vi "Get_Each_channel_reference_samplingdata.vi"(0 "SPU":refnum<k24>, 1 "STSProcess.ILSTS":refnum<k24>, 2 "Refdata_struct":refnum<k24>[](array[refnum]), 5 "Ref_monitordata_struct":refnum<k24>[](array[refnum]), 7 "MPM":refnum<k24>[](array[refnum]), 9 "ChannelNumber":i32, 11 "错误输入（无错误）":errorcluster, 12 "TSL":refnum<k24>, 13 "SlotNumber":i32, 14 "MPMNumber":i32) -> (6 "ILSTS out":refnum<k24>, 15 "error out":errorcluster)   [LabVIEW 2017]
doc: "Get logging reference data & add in"
uses:
  D:/test/ILSTS/LV_IL/LV_IL_Sample_x86/DLL/STSProcess.dll
  DLL/STSProcess.dll
  D:/test/ILSTS/LV_IL/LV_IL_Sample_x86/DLL/InstrumentDLL.dll
  DLL/InstrumentDLL.dll
  Share/PowerMonitorType.vi
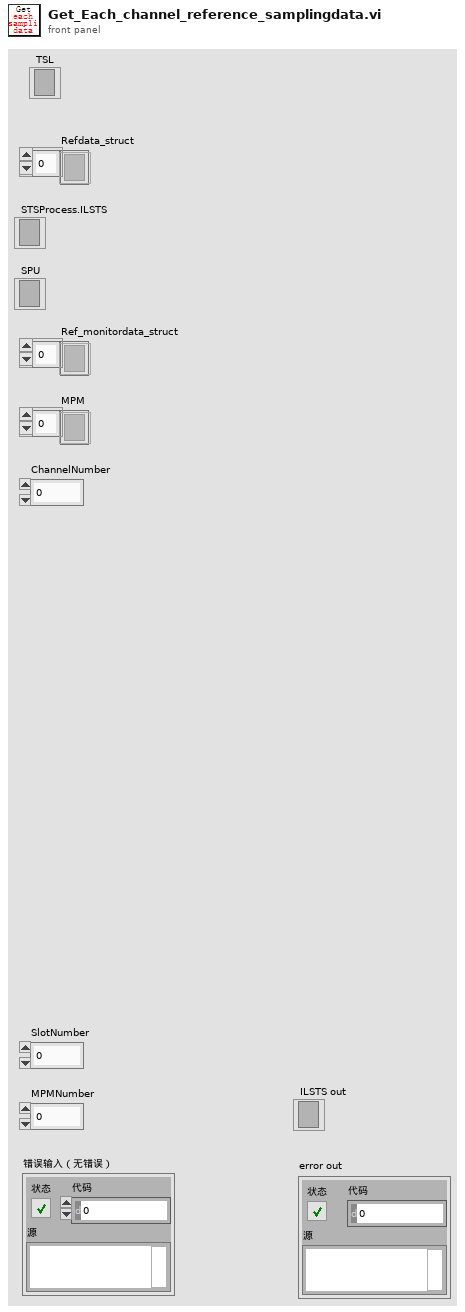
[diagram p1: front panel]
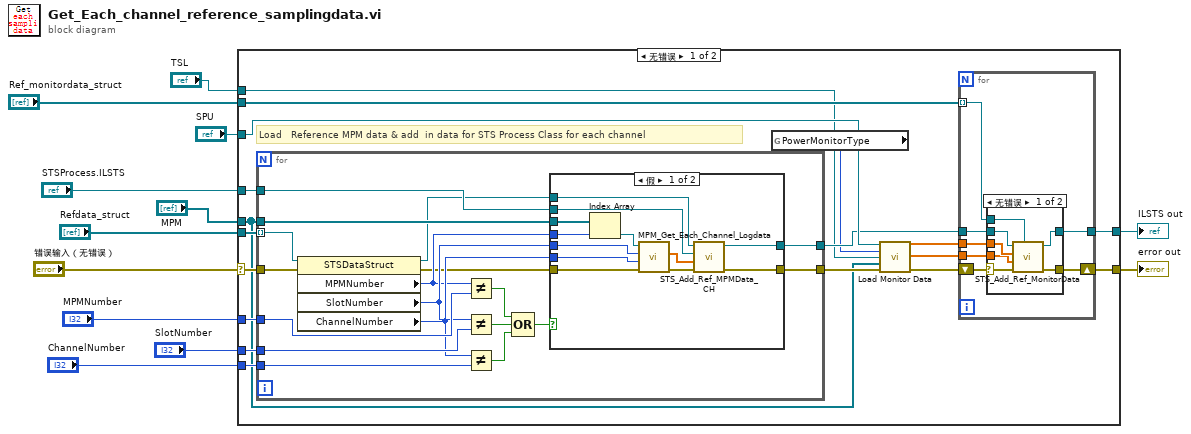
[diagram p0: block diagram]
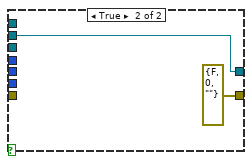
[diagram p3: hidden frame]
diagram:
  n1 = case shown="无错误" "错误输入（无错误）" {
    selector: "错误输入（无错误）" -> [w19 w80]
    tunnel: "STSProcess.ILSTS" -> [w17 w79]
    tunnel: "Ref_monitordata_struct" -> [w27 _]
    tunnel: "SPU" -> [w26 _]
    tunnel: "MPM" -> [w13 _]
    tunnel: "ChannelNumber" -> [w24 _]
    tunnel: "SlotNumber" -> [w23 _]
    tunnel: "MPMNumber" -> [w22 _]
    tunnel: "Refdata_struct" -> [w21 _]
    tunnel: [w20 w80] -> w4
    tunnel: [w18 w79] -> w2
    tunnel: "TSL" -> [w14 _]
    frame No Error {
      # "Load　Reference MPM data & add  in data for STS Process Class for each channel"
      n2 = for {
        tunnel: w21 -> [w52] mode=indexing
        tunnel: w22 -> [w64]
        tunnel: w23 -> [w63]
        tunnel: w24 -> [w62]
        tunnel: w13 -> [w55]
        tunnel: w17 -> [w53]
        tunnel: [w51] -> w25
        tunnel: w19 -> [w49]
        tunnel: [w47] -> w16
        n3 = property on="属性节点" class="STSDataStruct"(reference=w52, error in=w49) -> (reference out=w48:refnum<k24>, error out=w50:errorcluster, "MPMNumber"=w54:i32, "SlotNumber"=w57:i32, "ChannelNumber"=w56:i32)
        n4 = Not Equal?(x=w54, y=w64) -> (x != y?=w61:bool)
        n5 = Not Equal?(x=w57, y=w63) -> (x != y?=w60:bool)
        n6 = Not Equal?(x=w56, y=w62) -> (x != y?=w59:bool)
        n7 = Compound Arithmetic op=OR ("复合运算")(w61, w60, w59) -> (w58:bool)
        n8 = case shown="假" w58 {
          tunnel: w57 -> [w76 _]
          tunnel: w56 -> [w75 _]
          tunnel: w55 -> [w74 _]
          tunnel: w54 -> [w72 _]
          tunnel: w53 -> [w71 w77]
          tunnel: w48 -> [w70 _]
          tunnel: [w67 errorcluster {"status"=FALSE, "code"=0, "source"=""} ("错误输出")] -> w51
          tunnel: w50 -> [w66 _]
          tunnel: [w65 w77] -> w47
          frame False {
            n9 = Index Array(array=w74, index=w72) -> (element=w73:refnum<k24>)
            n10 = call "MPM_Get_Each_Channel_Logdata.vi"("error in (no error)"=w66, "channelNumber"=w75, "moduleNumber"=w76, ".NET Reference in"=w73) -> ("error out"=w68:errorcluster, "data out"=w69:sgl[])  [unwired: 5 in, 1 out]
            n11 = call "STS_Add_Ref_MPMData_CH.vi"("错误输入（无错误）"=w68, "data"=w69, "STSProcess.ILSTS"=w71, "Setting"=w70) -> ("错误输出"=w67:errorcluster, "ILSTS"=w65:refnum<k24>)  [unwired: 6 in]
          }
          frame True {
          }
        }
      }
      n12 = global read "PowerMonitorType.vi" "PowerMonitorType"() -> (w15:enum16{"DAQ", "MPM_220", "TSL_LOGG"})
      n13 = call "Load Monitor Data.vi"("SPU"=w26, "PowerMonitorType"=w15, "TSL"=w14, "MPM"=w13, "error in (no error)"=w25) -> ("trigger"=w29:sgl[], "monitor"=w30:sgl[], "error out"=w28:errorcluster)  [unwired: 8 in]
      n14 = for {
        tunnel: w27 -> [w36] mode=indexing
        tunnel: w16 -> [w37]
        tunnel: w29 -> [w35]
        tunnel: w30 -> [w34]
        shift-right: [w32] -> w20
        shift-left: w28 -> [w33]
        tunnel: [w31] -> w18
        n15 = case shown="无错误" w33 {
          selector: w33 -> [w40 w46]
          tunnel: w37 -> [w44 w45]
          tunnel: w36 -> [w43 _]
          tunnel: w35 -> [w42 _]
          tunnel: w34 -> [w41 _]
          tunnel: [w39 w46] -> w32
          tunnel: [w38 w45] -> w31
          frame No Error {
            n16 = call "STS_Add_Ref_MonitorData.vi"("setting"=w43, "错误输入（无错误）"=w40, "monitorData"=w41, "triggerIndex"=w42, "STSProcess.ILSTS"=w44) -> ("错误输出"=w39:errorcluster, "ILSTS out"=w38:refnum<k24>)  [unwired: 5 in]
          }
          frame Error {
          }
        }
      }
    }
    frame Error {
    }
  }
  "error out" <- w4
  "ILSTS out" <- w2
